vi "Actuator settings dialog.vi"(8 "error in (no error)":errorcluster) -> (0 "error out":errorcluster, 3 "Cancelled?":bool)   [LabVIEW 2016]
uses:
  Controls/Actuator fgv modes.ctl
panel:
  in  "COM port":refnum<visa-resource-name>
  in  "Confirm":bool
  in  "Cancel":bool
  # "ACTUATOR SETTINGS"
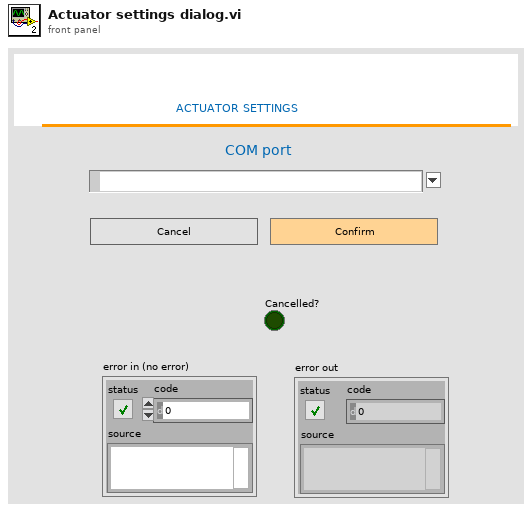
[diagram p1: front panel]
types:
  T1 = typedef "Actuator fgv modes.ctl" = enum16{"Initalise", "COM", "Limit", "Speed", "Home", "Get"}
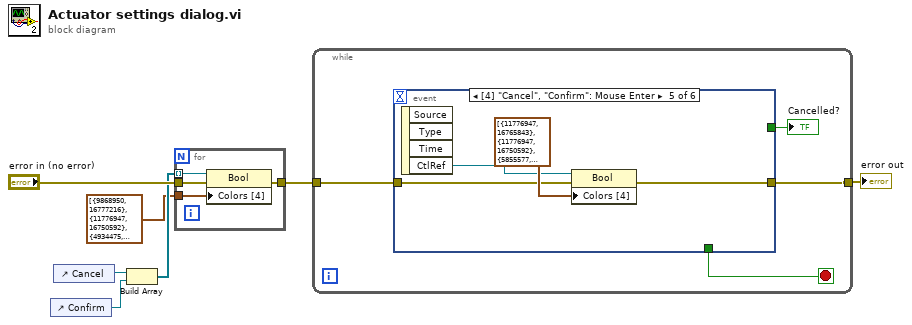
[diagram p0: block diagram]
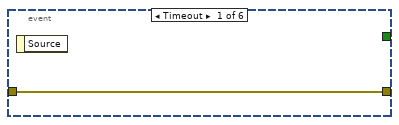
[diagram p2: hidden frame]
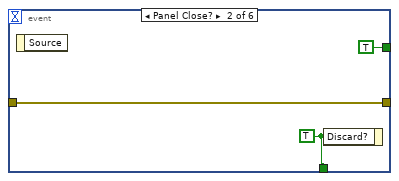
[diagram p3: hidden frame]
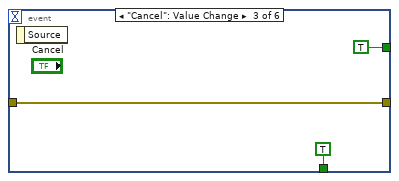
[diagram p4: hidden frame]
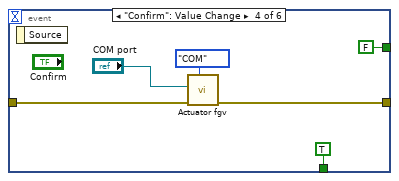
[diagram p5: hidden frame]
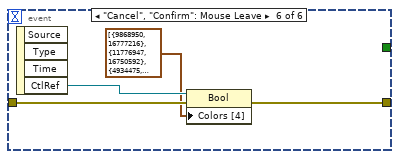
[diagram p6: hidden frame]
diagram:
  n1 = control-ref of="Confirm"() -> (w5:refnum<vi>)
  n2 = control-ref of="Cancel"() -> (w6:refnum<vi>)
  n3 = Build Array(w6, w5) -> (w3:refnum<vi>[])
  n4 = for {
    tunnel: "error in (no error)" -> [w11]
    tunnel: [w10] -> w1
    tunnel: w3 -> [w9] mode=indexing
    tunnel: cluster{u32, u32}[] [{9868950, 16777216}, {11776947, 16750592}, {4934475, 16777216}, {5855577, 8342528}] ("Colors [4]") -> [w8]
    n5 = property class="Bool"(reference=w9, error in=w11, "Colors [4]"=w8) -> (error out=w10:errorcluster)  [unwired: 1 out]
  }
  n6 = while {
    tunnel: w1 -> [w14]
    tunnel: [w13] -> w7
    stop <- w15 stop-if-true
    n7 = event shown="[4] \"Cancel\", \"Confirm\": Mouse Enter" {
      selector: _ -> [_ _ _ _ _ _]
      dyn-events: _ -> [_ _ _ _ _ _]
      timeout: _ -> [_ _ _ _ _ _]
      tunnel: [_ w19 TRUE ("Discard?") TRUE ("Discard?") _ _] -> w15
      tunnel: w14 -> [w16 w18 w21 w27 w31 w36]
      tunnel: [w16 w18 w21 w26 w30 w35] -> w13
      tunnel: [_ TRUE TRUE FALSE _ _] -> w12
      event Timeout {
        n8 = event-data() -> ()  [unwired: 1 in, 1 out]
      }
      event Panel Close? {
        w19 = TRUE ("Discard?")
        n9 = event-data() -> ()  [unwired: 1 in, 1 out]
        n10 = event-data("Discard?"=w19) -> ()  [unwired: 1 in, 1 out]
      }
      event "Cancel": Value Change {
        n11 = event-data() -> ()  [unwired: 1 in, 1 out]
      }
      event "Confirm": Value Change {
        n12 = event-data() -> ()  [unwired: 1 in, 1 out]
        n13 = call "Actuator fgv.vi"("Enum"=Actuator_fgv_modes."COM", "error in (no error)"=w27, "Data"="COM port") -> ("error out"=w26:errorcluster)  [unwired: 7 in, 1 out]
      }
      event "Cancel", "Confirm": Mouse Enter {
        n14 = event-data() -> ("CtlRef"=w29:refnum<vi>)  [unwired: 1 in, 3 out]
        n15 = property class="Bool"(reference=w29, error in=w31, "Colors [4]"=cluster{u32, u32}[] [{11776947, 16765843}, {11776947, 16750592}, {5855577, 8350025}, {5855577, 8342528}]) -> (error out=w30:errorcluster)  [unwired: 1 out]
      }
      event "Cancel", "Confirm": Mouse Leave {
        n16 = event-data() -> ("CtlRef"=w34:refnum<vi>)  [unwired: 1 in, 3 out]
        n17 = property class="Bool"(reference=w34, error in=w36, "Colors [4]"=cluster{u32, u32}[] [{9868950, 16777216}, {11776947, 16750592}, {4934475, 16777216}, {5855577, 8342528}]) -> (error out=w35:errorcluster)  [unwired: 1 out]
      }
    }
    "Cancelled?" <- w12
  }
  "error out" <- w7
